vi "MFLIcontrol.vi"(6 "SigIns0 Autorange":bool, 7 "Value":dbl, 8 "error in":errorcluster, 10 "MFLI function":T2, 11 "handle in":T3 {"Handle" format="0x%08x"; "Conn" format="0x%08x"}) -> (0 "error out":errorcluster, 1 "Demod Sample Out 2":T1={"Timestamps (ticks)"=0, "X (Vrms)"=nan, "Y (Vrms)"=nan, "Osc Phase (deg)"=nan, "Freq (Hz)"=nan, "DIO"=0, "AuxIn0 (V)"=nan, "AuxIn1 (V)"=nan, "Trigger"=0}, 2 "Demod Sample Out 3":T1={"Timestamps (ticks)"=0, "X (Vrms)"=nan, "Y (Vrms)"=nan, "Osc Phase (deg)"=nan, "Freq (Hz)"=nan, "DIO"=0, "AuxIn0 (V)"=nan, "AuxIn1 (V)"=nan, "Trigger"=0}, 3 "handle out":T3 {"Handle" format="0x%08x"; "Conn" format="0x%08x"})   [LabVIEW 2017]
uses:
  <instrlib>/Zurich Instruments LabOne/Public/ziTypeHandle.ctl
  MFLIcommand.ctl
  <instrlib>/Zurich Instruments LabOne/Public/Data/ziTypeDemodSampleSingle.ctl
  <instrlib>/Zurich Instruments LabOne/Public/Configure/ziGetValueDemodSampleEx.vi
  <instrlib>/Zurich Instruments LabOne/Public/Configure/ziSetValueDouble.vi
  <instrlib>/Zurich Instruments LabOne/Zurich Instruments LabOne.lvlib
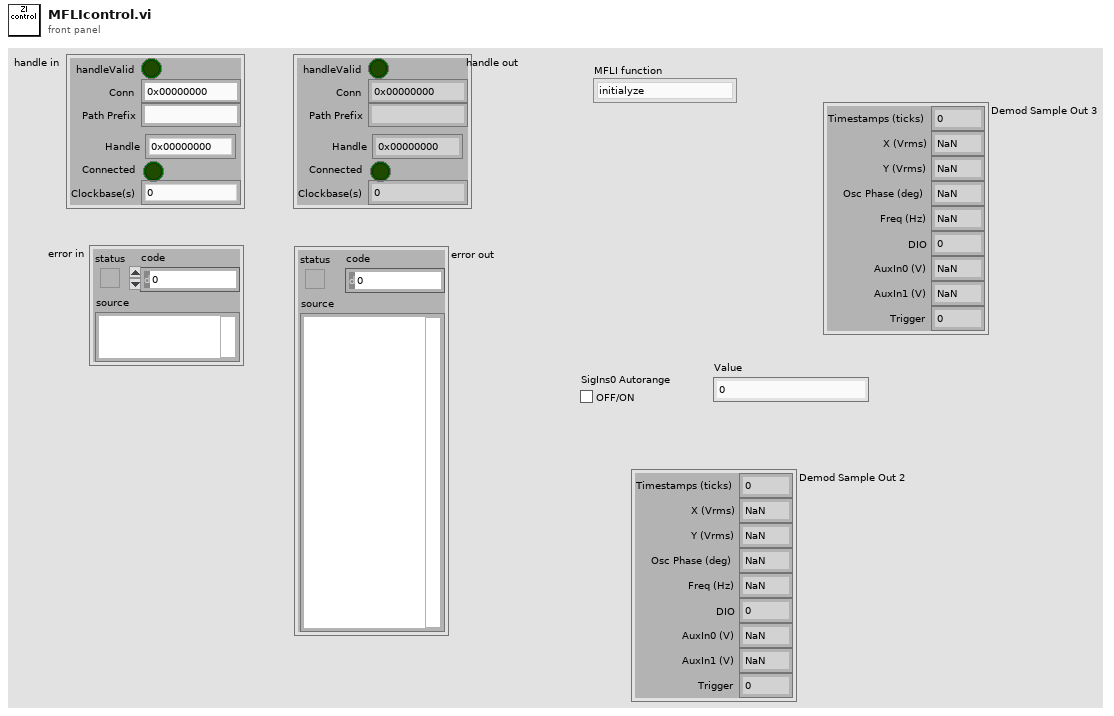
[diagram p1: front panel]
types:
  T1 = typedef "Zurich Instruments LabOne.lvlib/ziTypeDemodSampleSingle.ctl" = cluster{"Timestamps (ticks)":u64, "X (Vrms)":dbl, "Y (Vrms)":dbl, "Osc Phase (deg)":dbl, "Freq (Hz)":dbl, "DIO":u32, "AuxIn0 (V)":dbl, "AuxIn1 (V)":dbl, "Trigger":u32}
  T2 = typedef "MFLIcommand.ctl" = enum16{"initialyze", "measure current", "measure XY on demod0", "Set AuxOut1", "Set AuxOut2", "Set AuxOut3", "Set AuxOut4", "Set Osc Ampl", "SigIns Autorange", "finalyze", "Set Osc1 Freq"}
  T3 = typedef "Zurich Instruments LabOne.lvlib/ziTypeHandle.ctl" = cluster{"handleValid":bool, "Conn":u64, "Path Prefix":string, "Handle":u64, "Connected":bool, "Clockbase(s)":dbl}
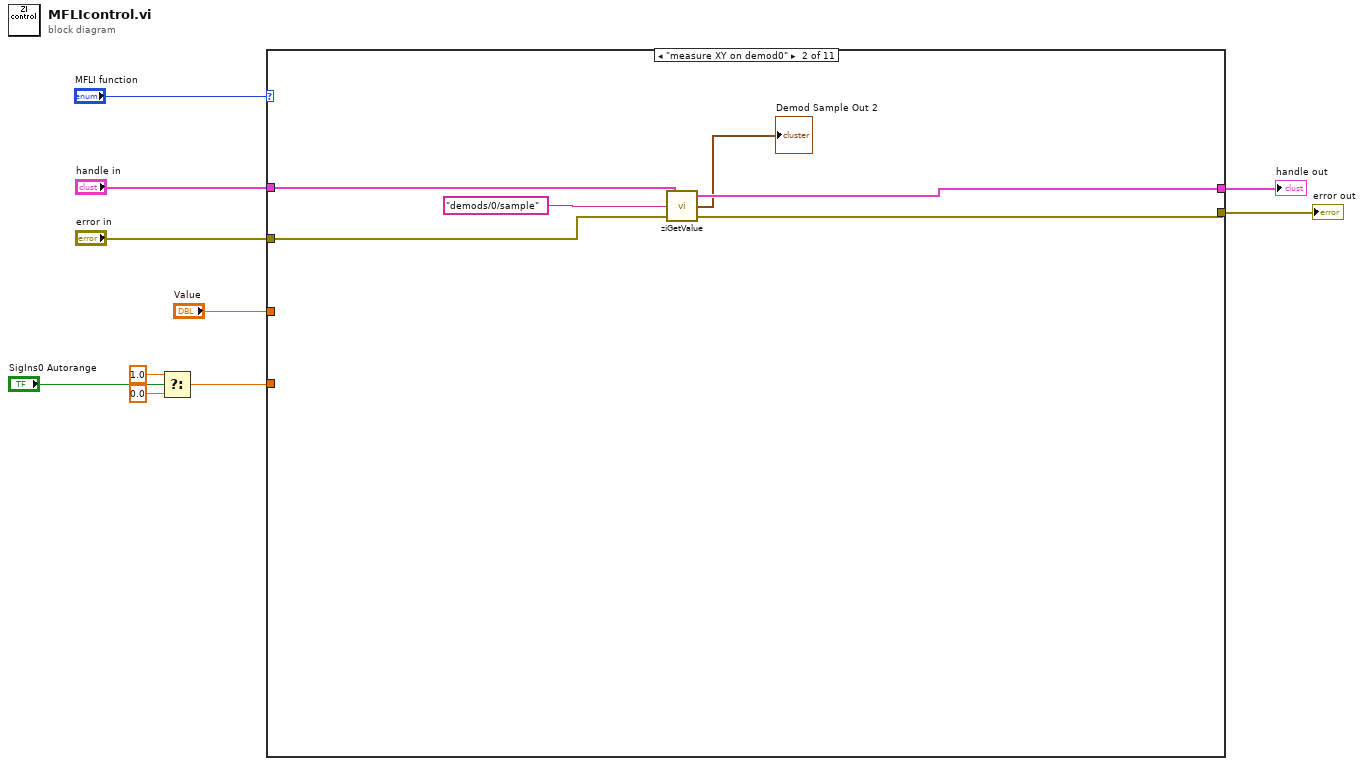
[diagram p0: block diagram]
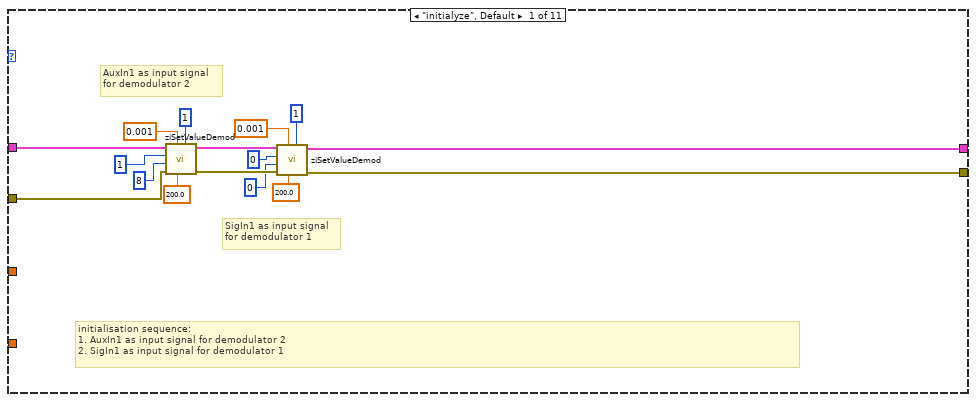
[diagram p2: hidden frame]
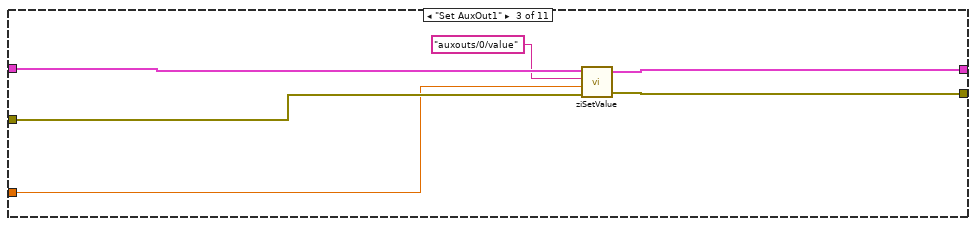
[diagram p3: hidden frame]
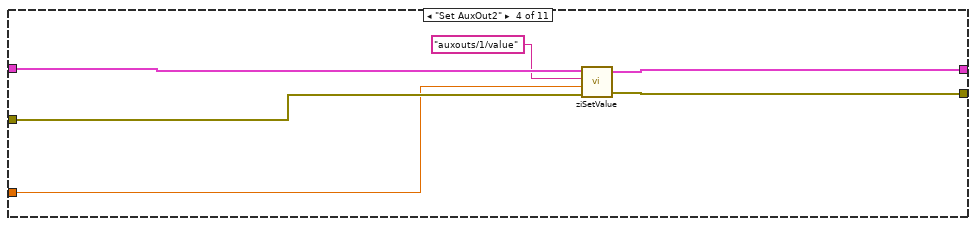
[diagram p4: hidden frame]
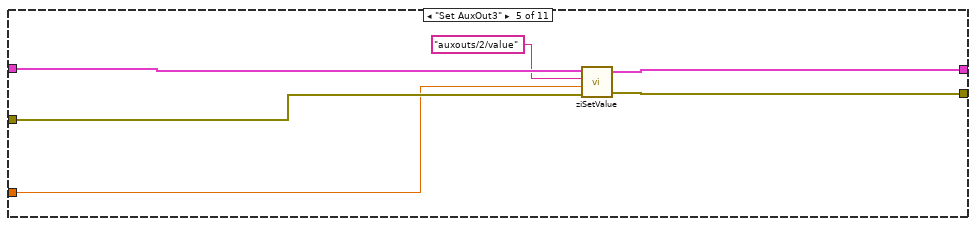
[diagram p5: hidden frame]
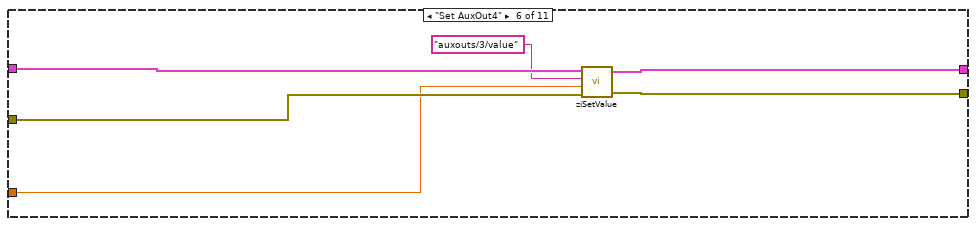
[diagram p6: hidden frame]
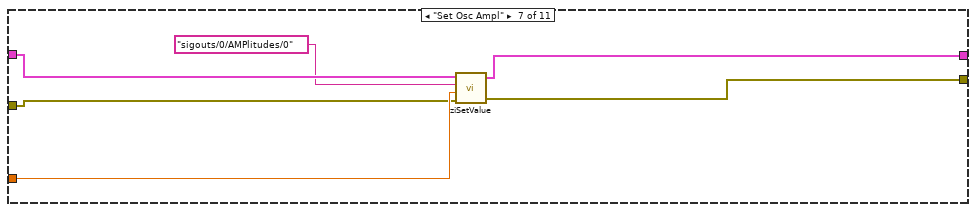
[diagram p7: hidden frame]
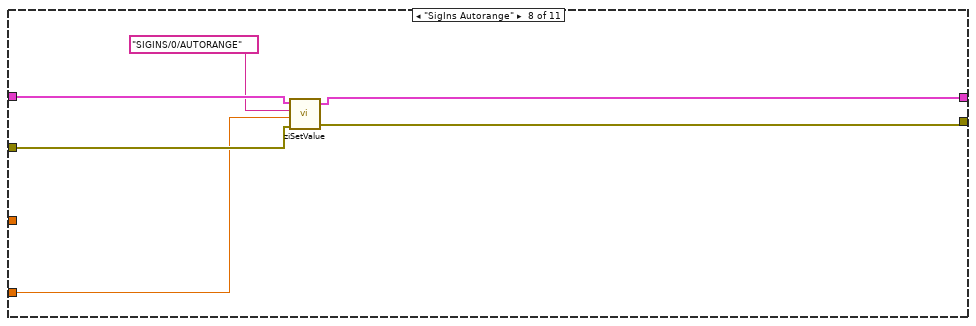
[diagram p8: hidden frame]
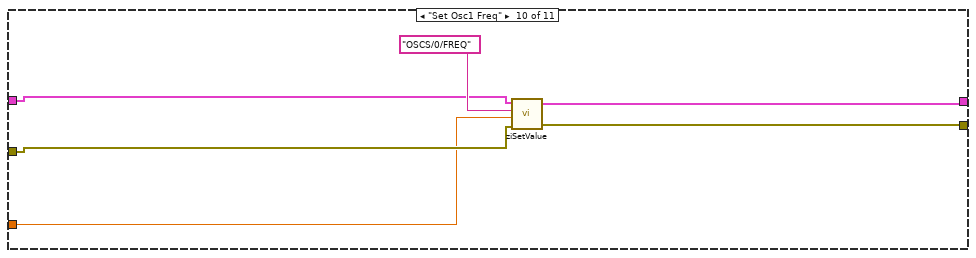
[diagram p10: hidden frame]
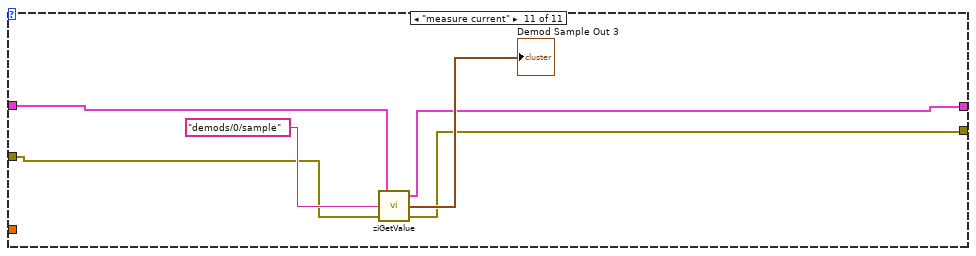
[diagram p11: hidden frame]
diagram:
  n1 = Select(t=1.0, s="SigIns0 Autorange", f=0.0) -> (s? t:f=w1:dbl)
  n2 = case shown="\"measure XY on demod0\"" "MFLI function" {
    tunnel: "handle in" -> [w26 w32 w38 w44 w50 w56 w62 w68 w70 w75 w80]
    tunnel: "error in" -> [w25 w30 w37 w43 w49 w55 w59 w67 w69 w74 w79]
    tunnel: [w24 w29 w36 w42 w48 w54 w58 w66 w70 w73 w78] -> w8
    tunnel: [w23 w28 w35 w41 w47 w53 w57 w65 w69 w72 w77] -> w7
    tunnel: "Value" -> [_ _ w33 w39 w45 w51 w60 _ _ w71 _]
    tunnel: w1 -> [_ _ _ _ _ _ _ w63 _ _ _]
    frame "initialyze", Default {
      # "initialisation sequence:\n1. AuxIn1 as input signal for demodulator 2 \n2. SigIn1 as input signal for demodulator 1"
      # "SigIn1 as input signal \nfor demodulator 1"
      # "AuxIn1 as input signal \nfor demodulator 2"
      n3 = call <instrlib>:"ziSetValueDemod.vi"("Order (2)"=1, "Rate (200Hz)"=200.0, "Time Constant (1ms)"=0.001, "error in"=w25, "Signal Input Select (0)"=8, "Demodulator # (0)"=1, "handle in"=w26) -> ("error out"=w16:errorcluster, "handle out"=w17:T3)  [unwired: 3 in]
      n4 = call <instrlib>:"ziSetValueDemod.vi"("Order (2)"=1, "Rate (200Hz)"=200.0, "Time Constant (1ms)"=0.001, "error in"=w16, "Signal Input Select (0)"=0, "Demodulator # (0)"=0, "handle in"=w17) -> ("error out"=w23:errorcluster, "handle out"=w24:T3)  [unwired: 3 in]
    }
    frame "measure XY on demod0" {
      n5 = call-poly <instrlib>:"ziGetValue.vi"("error in"=w30, "Path"="demods/0/sample", "Handle In"=w32) -> ("error out"=w28:errorcluster, "Demod Sample Out"=→"Demod Sample Out 2":T1, "Handle Out"=w29:T3)
    }
    frame "Set AuxOut1" {
      n6 = call-poly <instrlib>:"ziSetValue.vi"("Error In"=w37, "Value"=w33, "Path"="auxouts/0/value", "Handle In"=w38) -> ("Error Out"=w35:errorcluster, "Handle Out"=w36:T3)  [unwired: 1 in]
    }
    frame "Set AuxOut2" {
      n7 = call-poly <instrlib>:"ziSetValue.vi"("Error In"=w43, "Value"=w39, "Path"="auxouts/1/value", "Handle In"=w44) -> ("Error Out"=w41:errorcluster, "Handle Out"=w42:T3)  [unwired: 1 in]
    }
    frame "Set AuxOut3" {
      n8 = call-poly <instrlib>:"ziSetValue.vi"("Error In"=w49, "Value"=w45, "Path"="auxouts/2/value", "Handle In"=w50) -> ("Error Out"=w47:errorcluster, "Handle Out"=w48:T3)  [unwired: 1 in]
    }
    frame "Set AuxOut4" {
      n9 = call-poly <instrlib>:"ziSetValue.vi"("Error In"=w55, "Value"=w51, "Path"="auxouts/3/value", "Handle In"=w56) -> ("Error Out"=w53:errorcluster, "Handle Out"=w54:T3)  [unwired: 1 in]
    }
    frame "Set Osc Ampl" {
      n10 = call-poly <instrlib>:"ziSetValue.vi"("Error In"=w59, "Value"=w60, "Path"="sigouts/0/AMPlitudes/0", "Handle In"=w62) -> ("Error Out"=w57:errorcluster, "Handle Out"=w58:T3)  [unwired: 1 in]
    }
    frame "SigIns Autorange" {
      n11 = call-poly <instrlib>:"ziSetValue.vi"("Error In"=w67, "Value"=w63, "Path"="SIGINS/0/AUTORANGE", "Handle In"=w68) -> ("Error Out"=w65:errorcluster, "Handle Out"=w66:T3)  [unwired: 1 in]
    }
    frame "finalyze" {
    }
    frame "Set Osc1 Freq" {
      n12 = call-poly <instrlib>:"ziSetValue.vi"("Error In"=w74, "Value"=w71, "Path"="OSCS/0/FREQ", "Handle In"=w75) -> ("Error Out"=w72:errorcluster, "Handle Out"=w73:T3)  [unwired: 1 in]
    }
    frame "measure current" {
      n13 = call-poly <instrlib>:"ziGetValue.vi"("error in"=w79, "Path"="demods/0/sample", "Handle In"=w80) -> ("error out"=w77:errorcluster, "Demod Sample Out"=→"Demod Sample Out 3":T1, "Handle Out"=w78:T3)
    }
  }
  "handle out" <- w8
  "error out" <- w7
